vi "intent_comunicaico.vi"() -> ()   [LabVIEW 2009]
panel:
  out "array":dbl[][](array[numeric])
  out "Array":dbl[][][](array[numeric])
  out "data out":string
  in  "id":i32
  in  "buffer":i32=300
  in  "number data":i32=1
  in  "Dada":i32
  in  "adreça":i32
  in  "command":i32
  in  "stop":bool
  in  "Send":bool
  out "data logged":string
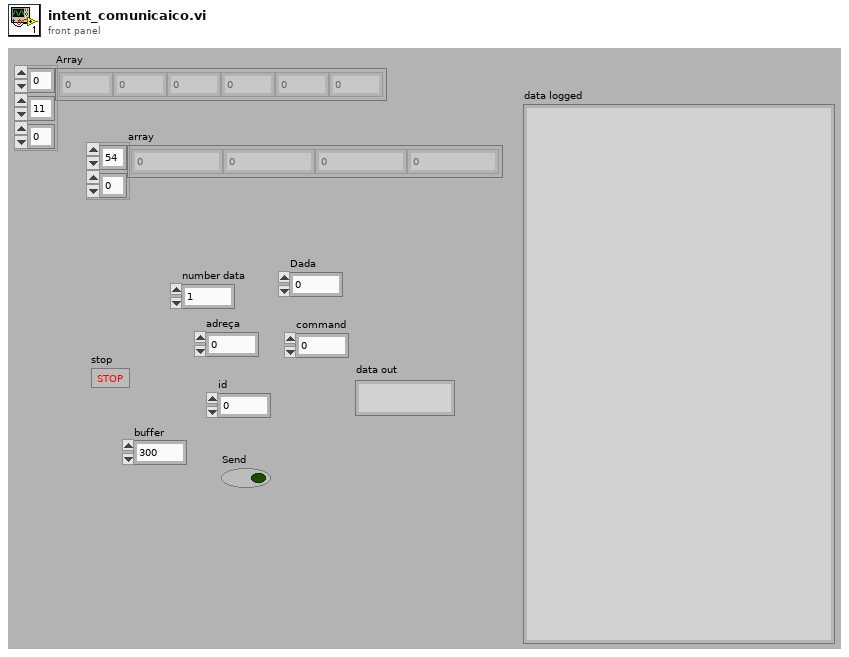
[diagram p1: front panel]
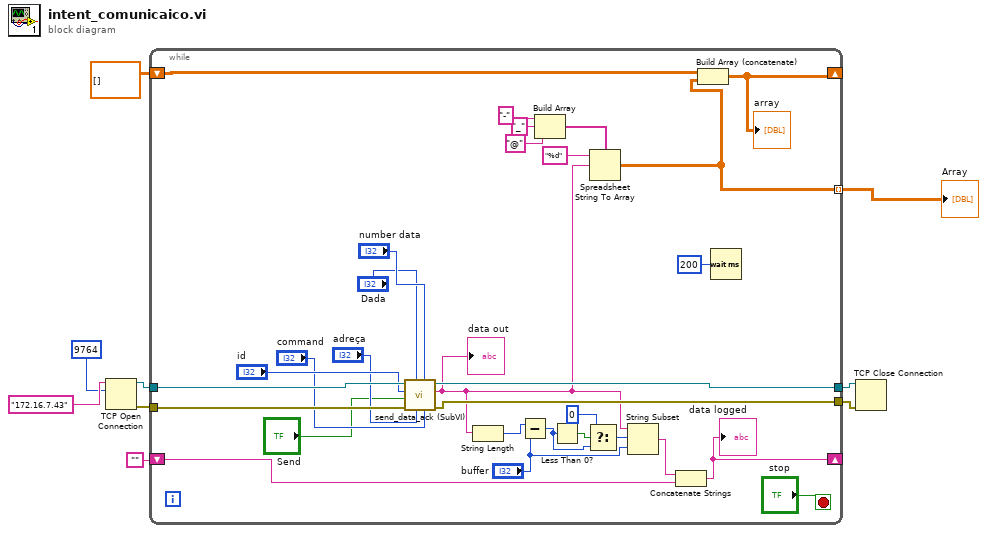
[diagram p0: block diagram]
diagram:
  n1 = TCP Open Connection(address="172.16.7.43", remote port or service name=u16 9764) -> (connection ID=w4:refnum<k5>, error out=w3:errorcluster)  [unwired: 3 in]
  n2 = while {
    shift-right: [w31] -> _
    shift-left: "" -> [w30]
    tunnel: [w29] -> w8
    tunnel: [w28] -> w7
    tunnel: w4 -> [w27]
    tunnel: w3 -> [w26]
    tunnel: [w14] -> w2 mode=indexing
    shift-right: [w12] -> _
    shift-left: dbl[][] [] -> [w13]
    stop <- "stop" stop-if-true
    n3 = call "send_data_ack (SubVI).vi"("command"="command", "number data"="number data", "adreça"="adreça", "Dada"="Dada", "error out"=w26, "Send"="Send", "id"="id", "connection ID"=w27) -> ("error out 2"=w28:errorcluster, "data out"=w20:string, "connection ID out"=w29:refnum<k5>)  [unwired: 1 out]
    "data out" <- w20
    n4 = String Length(string=w20) -> (length=w38:i32)
    n5 = Subtract(x=w38, y="buffer") -> (x-y=w35:i32)
    n6 = Build Array("-" ("spreadsheet string"), "_" ("element"), "@" ("element")) -> (w18:string[])
    n7 = Less Than 0?(x=w35) -> (x < 0?=w37:bool)
    n8 = Select(t=0, s=w37, f=w35) -> (s? t:f=w34:i32)
    n9 = Spreadsheet String To Array(delimiter (Tab)=w18, format string="%d", spreadsheet string=w20) -> (array=w14:dbl[][])  [unwired: 1 in]
    n10 = String Subset(string=w20, offset (0)=w34, length (rest)="buffer") -> (substring=w32:string)
    n11 = Concatenate Strings(w32, w30) -> (w31:string)
    "data logged" <- w31
    n12 = Build Array (concatenate)(w13, w14) -> (w12:dbl[][])
    "array" <- w12
    n13 = Wait (ms)(milliseconds to wait=u32 200) -> ()  [unwired: 1 out]
  }
  "Array" <- w2
  n14 = TCP Close Connection(connection ID=w8, error in (no error)=w7) -> ()  [unwired: 1 in, 2 out]
